vi "Get array index (Write to JSON).vi"(0 "Single element name":string, 5 "previous\n level\n cluster":variant, 9 "Object name":string, 11 "error in (no error)":errorcluster) -> (4 "index out":i32, 6 "key":string, 8 "VArray":variant, 10 "value":string, 13 "Element Present?":bool, 14 "Array Present?":bool, 15 "error out":errorcluster)   [LabVIEW 2015]
uses:
  <vilib>/regexp/Match Regular Expression.xnode
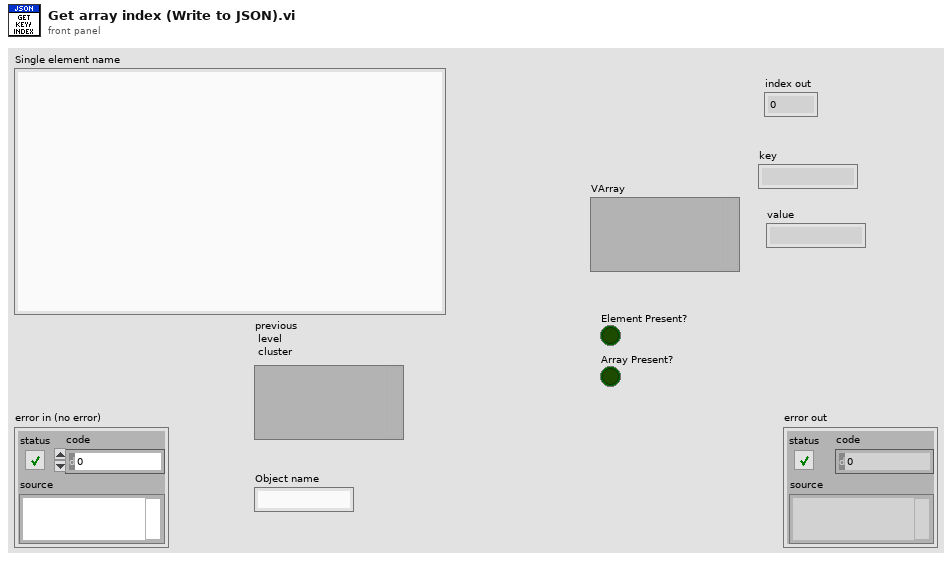
[diagram p1: front panel]
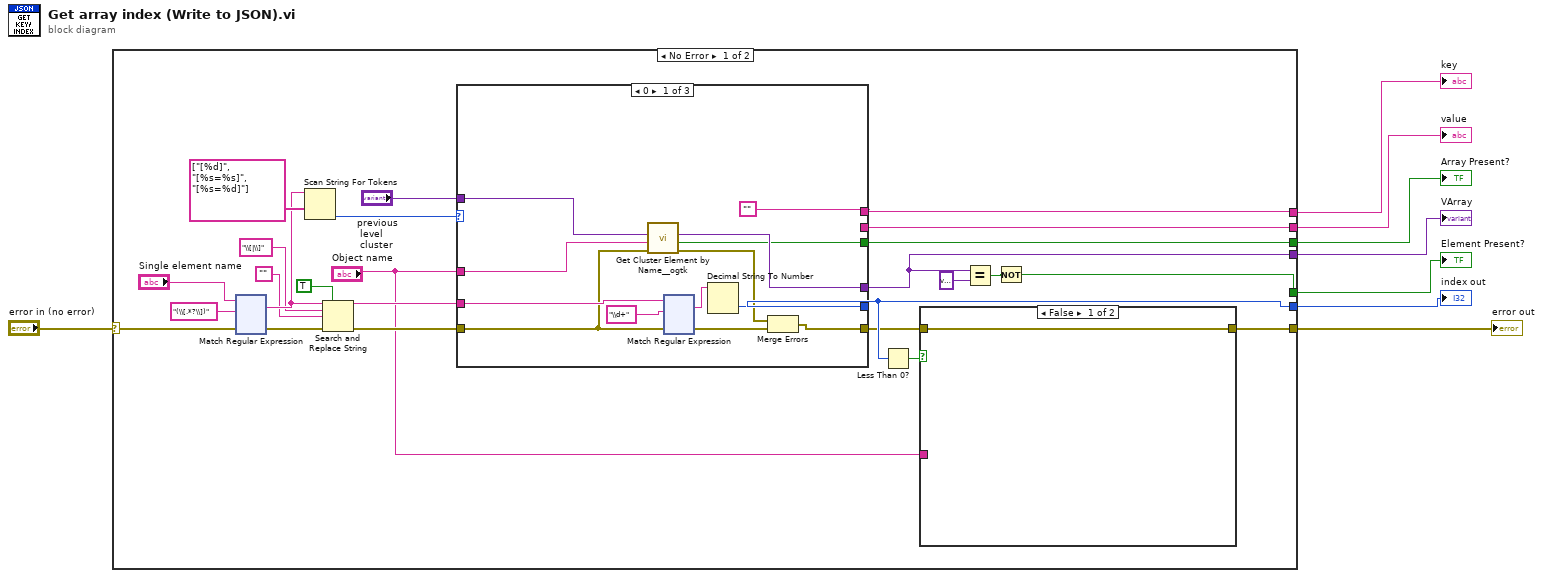
[diagram p0: block diagram]
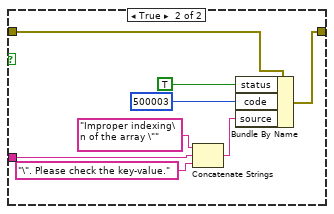
[diagram p2: hidden frame]
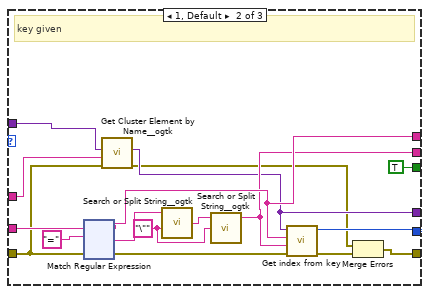
[diagram p3: hidden frame]
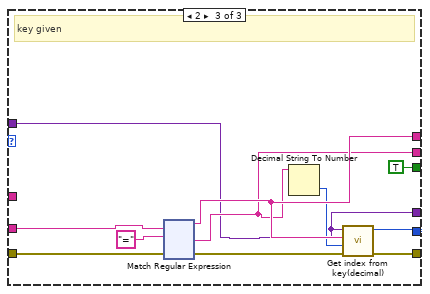
[diagram p4: hidden frame]
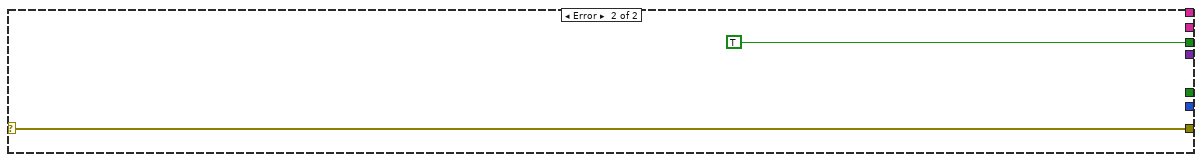
[diagram p5: hidden frame]
diagram:
  n1 = case shown="No Error" "error in (no error)" {
    selector: "error in (no error)" -> [w22 w541]
    tunnel: [w12 w541] -> w7
    tunnel: [w13 _] -> w6
    tunnel: [w21 _] -> w5
    tunnel: [w20 _] -> w4
    tunnel: [w18 TRUE ("found?")] -> w3
    tunnel: [w14 _] -> w2
    tunnel: [w15 _] -> w1
    frame No Error {
      n2 = xnode "Match Regular Expression"("input string"="Single element name", "regular expression"="(\\[.*?\\])", "error in"=w22) -> ("whole match"=w30:string, "error out"=w23:errorcluster)  [unwired: 3 in, 3 out]
      n3 = Scan String For Tokens(7:string[] ["[%d]", "[%s=%s]", "[%s=%d]"] ("operators (none)"), 9:w30) -> (0:w25:i32)  [unwired: 4 in, 3 out]
      n4 = Search and Replace String(replace all?=TRUE ("replace all? (F)"), input string=w30, search string="\\[|\\]", replace string="", error in=w23) -> (result string=w27:string, error out=w24:errorcluster)  [unwired: 3 in, 2 out]
      n5 = case shown="0" w25 {
        tunnel: w27 -> [w55 w186 w311]
        tunnel: w24 -> [w46 w176 w309]
        tunnel: [w52 w185 w308] -> w13
        tunnel: [w44 w170 w307] -> w11
        tunnel: [w51 w184 w306] -> w21
        tunnel: [w51 w177 w305] -> w20
        tunnel: [w48 w173 w303] -> w14
        tunnel: "Object name" -> [w49 w174 _]
        tunnel: "previous\n level\n cluster" -> [w50 w175 w303]
        tunnel: [w47 TRUE ("found?") TRUE ("found?")] -> w18
        frame 0 {
          w51 = ""
          n6 = call <userlib>:"Get Cluster Element by Name__ogtk.vi"("error in (no error)"=w46, "Element Name"=w49, "Cluster"=w50) -> ("error out"=w43:errorcluster, "found?"=w47:bool, "VElement"=w48:variant)  [unwired: 6 in]
          n7 = xnode "Match Regular Expression"("input string"=w55, "regular expression"="\\d+", "error in"=w46) -> ("whole match"=w53:string, "error out"=w45:errorcluster)  [unwired: 3 in, 3 out]
          n8 = Decimal String To Number(string=w53) -> (number=w52:i32)  [unwired: 2 in, 1 out]
          n9 = Merge Errors(w43, w45) -> (w44:errorcluster)
        }
        frame 1, Default {
          w179 = "\"" ("search string/char (-)")
          # "key given"
          n10 = xnode "Match Regular Expression"("input string"=w186, "regular expression"="=", "error in"=w176) -> ("before match"=w184:string, "after match"=w178:string, "error out"=w182:errorcluster)  [unwired: 3 in, 2 out]
          n11 = call <userlib>:"Get Cluster Element by Name__ogtk.vi"("error in (no error)"=w176, "Element Name"=w174, "Cluster"=w175) -> ("error out"=w171:errorcluster, "VElement"=w173:variant)  [unwired: 6 in, 1 out]
          n12 = call <userlib>:"Search or Split String__ogtk.vi"("search string/char (-)"=w179, "string"=w178) -> ("substring after match"=w180:string)  [unwired: 1 in, 2 out]
          n13 = call <userlib>:"Search or Split String__ogtk.vi"("search string/char (-)"=w179, "string"=w180) -> ("substring before match"=w177:string)  [unwired: 1 in, 2 out]
          n14 = call "Get index from key.vi"("error in (no error)"=w182, "value"=w177, "key"=w184, "VElement"=w173) -> ("error out"=w172:errorcluster, "indexOut"=w185:i32)  [unwired: 6 in]
          n15 = Merge Errors(w171, w172) -> (w170:errorcluster)
        }
        frame 2 {
          # "key given"
          n16 = xnode "Match Regular Expression"("input string"=w311, "regular expression"="=", "error in"=w309) -> ("before match"=w306:string, "after match"=w305:string, "error out"=w302:errorcluster)  [unwired: 3 in, 2 out]
          n17 = Decimal String To Number(string=w305) -> (number=w304:i32)  [unwired: 2 in, 1 out]
          n18 = call "Get index from key(decimal).vi"("error in (no error)"=w302, "Value(decimal)"=w304, "key"=w306, "VElement"=w303) -> ("error out"=w307:errorcluster, "indexOut"=w308:i32)  [unwired: 6 in]
        }
      }
      n19 = Less Than 0?(x=w13) -> (x < 0?=w10:bool)
      n20 = case shown="False" w10 {
        tunnel: [w34 w39] -> w12
        tunnel: w11 -> [w34 w42]
        tunnel: "Object name" -> [_ w37]
        frame False {
        }
        frame True {
          n21 = Concatenate Strings("Improper indexing\n of the array \"" ("source"), w37, "\". Please check the key-value." ("string")) -> (w35:string)
          n22 = Bundle By Name(cluster=w42, "status"=TRUE, "code"=500003, "source"=w35) -> (w39:errorcluster)
        }
      }
      n23 = Equal?(x=w14, y=variant) -> (x = y?=w16:bool)
      n24 = Not(x=w16) -> (.not. x?=w15:bool)
    }
    frame Error {
    }
  }
  "error out" <- w7
  "index out" <- w6
  "key" <- w5
  "value" <- w4
  "Array Present?" <- w3
  "VArray" <- w2
  "Element Present?" <- w1
